vi "Get(path).vi"(8 "error in (no error)":errorcluster, 10 "Path":string, 11 "JSON Value in":refnum<class "JSON Value.lvclass">) -> (0 "error out":errorcluster, 2 "JSON Value out":refnum<class "JSON Value.lvclass">, 3 "JSON Value out":refnum<class "JSON Value.lvclass">)   [LabVIEW 2016, in "JSON Value.lvclass"]
uses:
  JSON Value.lvclass
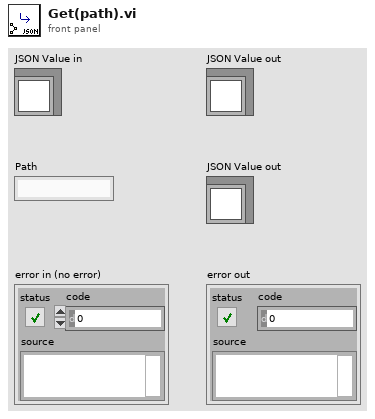
[diagram p1: front panel]
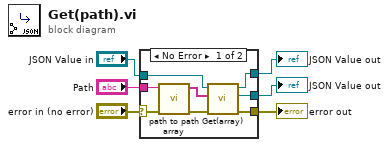
[diagram p0: block diagram]
diagram:
  n1 = case shown="No Error" "error in (no error)" {
    selector: "error in (no error)" -> [w13 w15]
    tunnel: "Path" -> [w14 _]
    tunnel: "JSON Value in" -> [w11 w16]
    tunnel: [w10 _] -> w3
    tunnel: [w9 w16] -> w2
    tunnel: [w7 w15] -> w1
    frame No Error {
      n2 = call "path to path array.vi"("error in (no error)"=w13, "path"=w14) -> ("error out"=w8:errorcluster, "path array"=w12:string[])  [unwired: 8 in]
      n3 = call "Get(array).vi"("error in (no error)"=w8, "Path Array"=w12, "JSON Value in"=w11) -> ("error out"=w7:errorcluster, 2:"JSON Value out"=w9:refnum<class "JSON Value.lvclass">, 3:"JSON Value out"=w10:refnum<class "JSON Value.lvclass">)  [unwired: 6 in]
    }
    frame Error {
    }
  }
  "JSON Value out" <- w3
  "error out" <- w1
  "JSON Value out" <- w2
